vi "toImmediate.vi"(11 "raise or lower arm":dbl) -> ()   [LabVIEW 2018]
uses:
  <vilib>/Rock Robotics/WPI/Framework/Command Status Info.ctl
  <vilib>/Rock Robotics/WPI/Framework/Completion Status.ctl
  <vilib>/Rock Robotics/WPI/Framework/Completion Notifier.ctl
  Implementation/Manipulator Setpoints.ctl
  Implementation/Manipulator Operations.ctl
panel:
  in  "Description":string="Reserve"
  in  "Command Name":string
  out "Command Info":T1
  in  "Command Info 2":T1
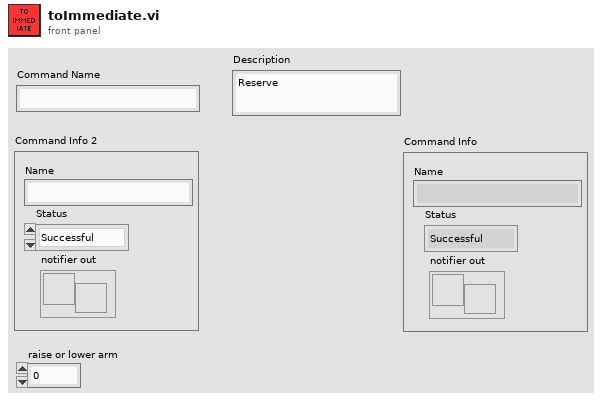
[diagram p1: front panel]
types:
  T1 = typedef "Command Status Info.ctl" = cluster{"Name":string, "Status":T2, "notifier out":T3}
  T2 = typedef "Completion Status.ctl" = enum16{"Successful", "Aborted", "Incomplete"}
  T3 = typedef "Completion Notifier.ctl" = refnum<notifier>
  T4 = typedef "Manipulator Setpoints.ctl" = cluster{"Operation":T5, "Setpoint":dbl, "Duration":dbl}
  T5 = typedef "Manipulator Operations.ctl" = enum16{"Reserve", "Read Current", "Immediate", "LowerArm", "RaiseArm", "HoldingCover"}
  T6 = cluster{"Operation":T5, "raise or lower arm":dbl, "Duration":dbl}
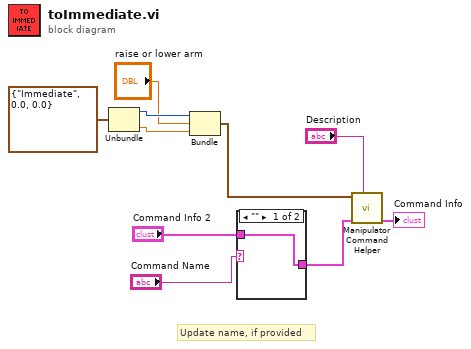
[diagram p0: block diagram]
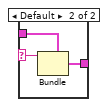
[diagram p2: hidden frame]
diagram:
  # "Update name, if provided"
  n1 = Unbundle(T4 {"Operation"=enum."Immediate", "Setpoint"=0.0, "Duration"=0.0} ("SubSystem Data")) -> ("Operation"=w4:T5, "Duration"=w3:dbl)  [unwired: 1 out]
  n2 = Bundle("Operation"=w4, "raise or lower arm"="raise or lower arm", "Duration"=w3) -> (w1:T6)  [unwired: 1 in]
  n3 = case shown="\"\"" "Command Name" {
    selector: "Command Name" -> [_ w12]
    tunnel: "Command Info 2" -> [w11 w14]
    tunnel: [w11 w13] -> w7
    frame "" {
    }
    frame Default {
      n4 = Bundle(cluster=w14, "Name"=w12) -> (w13:T1)  [unwired: 2 in]
    }
  }
  n5 = call "Manipulator Command Helper.vi"("Description"="Description", "Command Info In"=w7, "SubSystem Data"=w1) -> ("Command Info Out"=→"Command Info":T1)  [unwired: 6 in, 2 out]
